vi "TDMS N Chan N Samp.vi"() -> ()   [LabVIEW 2014]
uses:
  <vilib>/DAQmx/create/channels.llb/DAQmx Create Channel (AI-Voltage-Basic).vi
  <vilib>/DAQmx/configure/timing.llb/DAQmx Timing (Sample Clock).vi
  <vilib>/DAQmx/read.llb/DAQmx Read (Analog 1D Wfm NChan NSamp).vi
panel:
  in  "operation (0:open)":T1(ring)=enum."create or replace"
  in  "file path":path
  in  "rate":dbl=1000.0 format="%0.2f"
  in  "physical channels":tag
  in  "Stop Button":bool
  # "Read Analog Channels and Write to TDMS Channels"
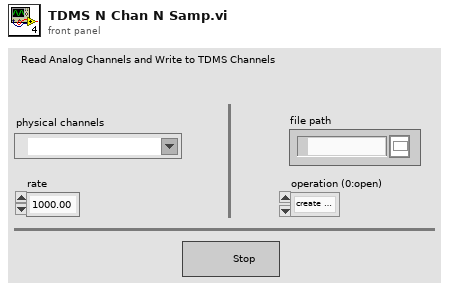
[diagram p1: front panel]
types:
  T1 = enum16{"open", "open or create", "create or replace", "create", "open (read-only)"}
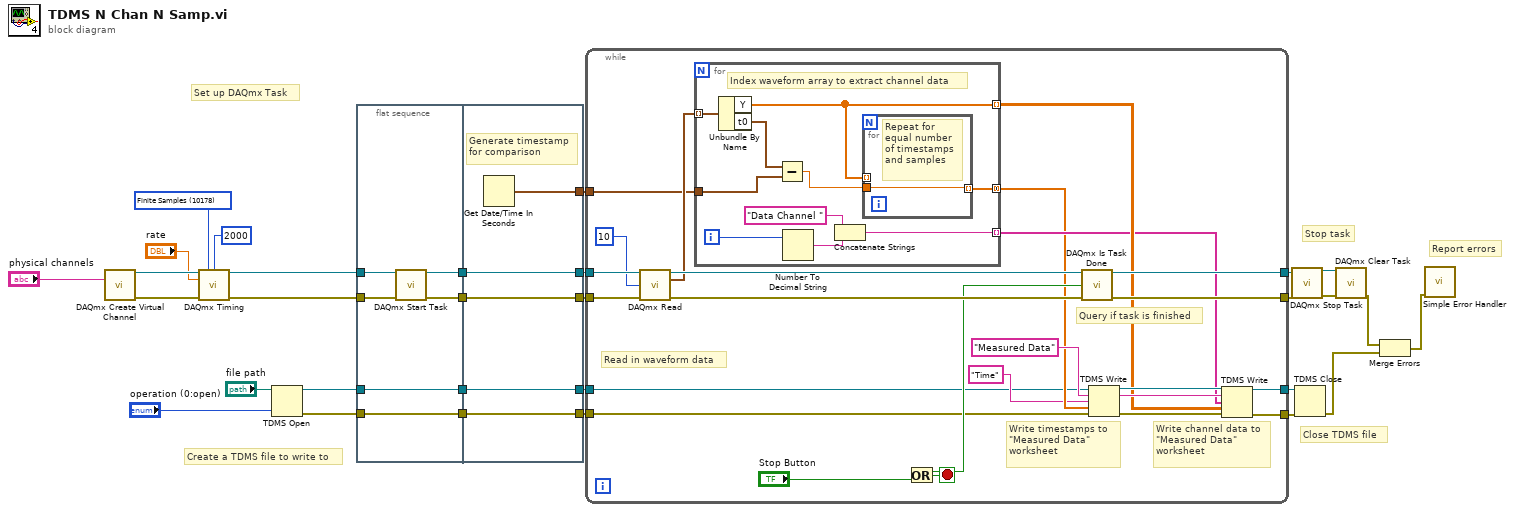
[diagram p0: block diagram]
diagram:
  w23 = 10178 items=["Finite Samples"=10178, "Continuous Samples"=10123, "Hardware Timed Single Point"=12522] ("sample mode")
  # "Report errors"
  # "Stop task"
  # "Close TDMS file"
  # "Create a TDMS file to write to"
  # "Set up DAQmx Task"
  n1 = call-poly <vilib>:"DAQmx Create Virtual Channel.vi"("physical channels"="physical channels") -> ("task out"=w30:refnum<k21>, "error out"=w29:errorcluster)  [unwired: 13 in]
  n2 = call-poly <vilib>:"DAQmx Timing.vi"("task/channels in"=w30, "sample mode"=w23, "samples per channel"=2000, "rate"="rate", "error in"=w29) -> ("task out"=w28:refnum<k21>, "error out"=w27:errorcluster)  [unwired: 9 in]
  n3 = TDMS Open(10:"operation (0:open)", 11:"file path") -> (0:w6:errorcluster, 3:w5:refnum<k34>)  [unwired: 5 in]
  n4 = flat-sequence {
    tunnel: w28 -> [w36]
    tunnel: w27 -> [w35]
    tunnel: [w34] -> w9
    tunnel: [w33] -> w8
    tunnel: w6 -> [w31]
    tunnel: w5 -> [w32]
    tunnel: [w32] -> w4
    tunnel: [w31] -> w3
    tunnel: [w40] -> w25
    tunnel: [w41] -> w26
    tunnel: w9 -> [w41]
    tunnel: w8 -> [w40]
    tunnel: [w39] -> w7
    tunnel: [w38] -> w1
    tunnel: w4 -> [w38]
    tunnel: w3 -> [w37]
    tunnel: [w37] -> w2
    frame #0 {
      n5 = call <vilib>:"DAQmx Start Task.vi"("task/channels in"=w36, "error in"=w35) -> ("task out"=w34:refnum<k21>, "error out"=w33:errorcluster)  [unwired: 12 in]
    }
    frame #1 {
      # "Generate timestamp\nfor comparison"
      n6 = Get Date/Time In Seconds() -> (seconds since 1Jan1904=w39:timestamp)
    }
  }
  n7 = while {
    tunnel: w26 -> [w59]
    tunnel: w25 -> [w58]
    tunnel: [w55] -> w21
    tunnel: [w51] -> w20
    tunnel: w7 -> [w49]
    tunnel: [w61] -> w15
    tunnel: [w60] -> w14
    tunnel: w2 -> [w43]
    tunnel: w1 -> [w42]
    stop <- w54 stop-if-true
    # "Query if task is finished"
    # "Write channel data to\n\"Measured Data\" \nworksheet"
    # "Write timestamps to \n\"Measured Data\" \nworksheet"
    # "Read in waveform data"
    n8 = call-poly <vilib>:"DAQmx Read.vi"("task/channels in"=w59, "number of samples per channel"=10, "error in"=w58) -> ("task out"=w57:refnum<k21>, "data"=w50:waveform(dbl)[], "error out"=w56:errorcluster)  [unwired: 10 in]
    n9 = for {
      tunnel: w50 -> [w75] mode=indexing
      tunnel: w49 -> [w73]
      tunnel: [w68] -> w48 mode=indexing
      tunnel: [w69] -> w47 mode=indexing
      tunnel: [w66] -> w45 mode=concatenating
      i -> [w70]
      # "Index waveform array to extract channel data"
      n10 = Unbundle By Name(w75) -> ("Y"=w68:dbl[], "t0"=w74:timestamp)
      n11 = Subtract(x=w74, y=w73) -> (x-y=w67:dbl)
      n12 = Number To Decimal String(number=w70) -> (decimal integer string=w71:string)  [unwired: 1 in]
      n13 = Concatenate Strings("Data Channel ", w71) -> (w69:string)
      n14 = for {
        tunnel: w68 -> [_] mode=indexing
        tunnel: w67 -> [w76]
        tunnel: [w76] -> w66 mode=indexing
        # "Repeat for\nequal number\nof timestamps\nand samples"
      }
    }
    n15 = call <vilib>:"DAQmx Is Task Done.vi"("task/channels in"=w57, "error in"=w56) -> ("task out"=w55:refnum<k21>, "task done?"=w52:bool, "error out"=w51:errorcluster)  [unwired: 11 in]
    n16 = Or(x=w52, y="Stop Button") -> (x .or. y?=w54:bool)
    n17 = TDMS Write(0:w42, 5:"Measured Data" ("group name in (Untitled)"), 7:"Time", 9:w45, 11:w43) -> (4:w64:refnum<k34>, 6:w62:string, 15:w63:errorcluster)  [unwired: 1 in, 1 out]
    n18 = TDMS Write(0:w64, 5:w62, 7:w47, 9:w48, 11:w63) -> (4:w61:refnum<k34>, 15:w60:errorcluster)  [unwired: 1 in, 2 out]
  }
  n19 = call <vilib>:"DAQmx Stop Task.vi"("task/channels in"=w21, "error in"=w20) -> ("task out"=w19:refnum<k21>, "error out"=w18:errorcluster)  [unwired: 12 in]
  n20 = TDMS Close(8:w14, 11:w15) -> (0:w11:errorcluster)  [unwired: 1 out]
  n21 = call <vilib>:"DAQmx Clear Task.vi"("task in"=w19, "error in"=w18) -> ("error out"=w13:errorcluster)  [unwired: 13 in]
  n22 = Merge Errors(w13, w11) -> (w12:errorcluster)
  n23 = call <vilib>:"Simple Error Handler.vi"("error in (no error)"=w12) -> ()  [unwired: 4 in, 5 out]
